vi "RSNRPZ One Sensor Connection.vi"(0 "Resource Name (USB::0xaad::0x00b::100000)":string="USB::0xaad::0x00b::100000", 5 "Reset Device (T: Reset Device)":bool=TRUE, 7 "ID Query (T: Do Query)":bool=TRUE, 9 "Correction Frequency ( 50.0e6 Hz)":dbl=50000000.0 format="%.2p", 11 "Timeout (10000 ms)":i32=10000) -> (6 "Measurement":dbl format="%.3p")   [LabVIEW 2010]
doc: "This VI runs one sensor measurement.\n- Open session to sensor specified by Resource Name\n- Sets correct frequency\n- Initialize acqusistion, wait specified time for measurement and reads it."
panel:
  # "NRP-Z Power Meter\nOne Sensor Measurement"
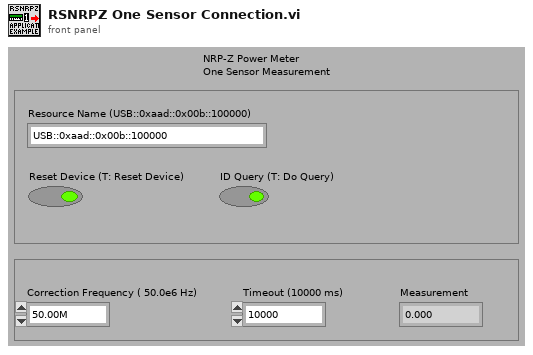
[diagram p1: front panel]
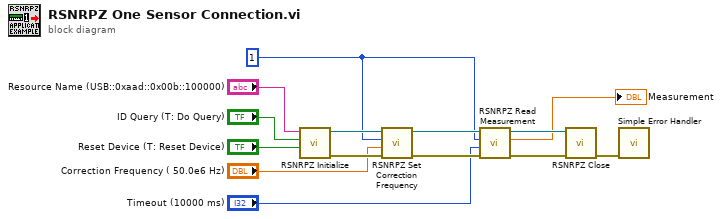
[diagram p0: block diagram]
diagram:
  w7 = 1 ("Channel (1)")
  n1 = call <instrlib>:"RSNRPZ Initialize.vi"("Reset Device (T: Reset Device)"="Reset Device (T: Reset Device)", "ID Query (T: Do Query)"="ID Query (T: Do Query)", "Resource Name (USB::0x0aad::0x000b::100000)"="Resource Name (USB::0xaad::0x00b::100000)") -> ("error out"=w13:errorcluster, "dup VISA session"=w14:refnum<visa-resource-name>)  [unwired: 7 in]
  n2 = call <instrlib>:"RSNRPZ Set Correction Frequency.vi"("error in (no error)"=w13, "Frequency ( 50.0e6 Hz)"="Correction Frequency ( 50.0e6 Hz)", "Channel (1)"=w7, "VISA session"=w14) -> ("error out"=w11:errorcluster, "dup VISA session"=w12:refnum<visa-resource-name>)  [unwired: 6 in]
  n3 = call <instrlib>:"RSNRPZ Read Measurement.vi"("error in (no error)"=w11, "Timeout (5000 ms)"="Timeout (10000 ms)", "Channel (1)"=w7, "VISA session"=w12) -> ("error out"=w2:errorcluster, "Measurement"=→"Measurement":dbl, "dup VISA session"=w10:refnum<visa-resource-name>)  [unwired: 5 in]
  n4 = call <instrlib>:"RSNRPZ Close.vi"("error in (no error)"=w2, "VISA session"=w10) -> ("error out"=w1:errorcluster)  [unwired: 9 in]
  n5 = call <vilib>:"Simple Error Handler.vi"("error in (no error)"=w1) -> ()  [unwired: 4 in, 5 out]
